vi "Main.vi"() -> ()   [LabVIEW 2009]
panel:
  out "data out":dbl[](array[numeric])
  in  "data in":dbl[](array[numeric])
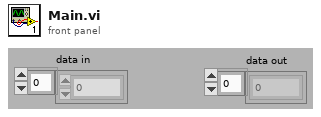
[diagram p1: front panel]
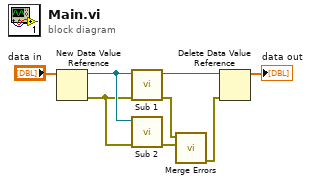
[diagram p0: block diagram]
diagram:
  n1 = New Data Value Reference(data value="data in") -> (data value reference=w7:refnum<data-value>, error out=w4:errorcluster)  [unwired: 1 in]
  n2 = call "Sub 1.vi"("error in (no error)"=w4, "data value reference"=w7) -> ("error out"=w3:errorcluster, "data value reference 2"=w6:refnum<data-value>)  [unwired: 8 in]
  n3 = call "Sub 2.vi"("error in (no error)"=w4, "data value reference"=w7) -> ("error out"=w2:errorcluster)  [unwired: 8 in, 1 out]
  n4 = call <vilib>:"Merge Errors.vi"("error in 2 (no error)"=w2, "error in 1 (no error)"=w3) -> ("error out"=w1:errorcluster)  [unwired: 5 in]
  n5 = Delete Data Value Reference(data value reference=w6, error in=w1) -> (data value=→"data out":dbl[])  [unwired: 1 out]
